vi "GetType.vi"(8 "error in (no error)":errorcluster, 11 "Control Mode Msg":refnum<class "Control Mode Msg.lvclass">) -> (0 "error out":errorcluster, 2 "Data Sample":variant, 3 "Control Mode Msg":refnum<class "Control Mode Msg.lvclass">)   [LabVIEW 2015, in "KIT-QVA.lvlib" / "Control Mode Msg.lvclass"]
doc: "This VI delivers a sample of the data type format the message expects."
uses:
  Control Mode Msg.lvclass
  Control Mode Msg.lvclass/Control Mode Msg.ctl
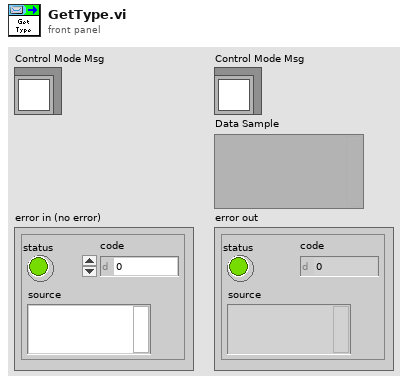
[diagram p1: front panel]
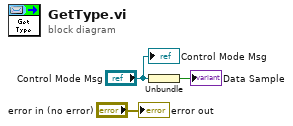
[diagram p0: block diagram]
diagram:
  n1 = Unbundle("Control Mode Msg") -> (→"Data Sample":bool)
  "error out" <- "error in (no error)"
  "Control Mode Msg" <- "Control Mode Msg"
